vi "re_1.vi"(1 "wait_ms":u32=1000) -> (0 "timer_ms":u32)   [LabVIEW 2015, in "lv_mutex_shared_1.lvlib"]
uses:
  lv_mutex_shared_1.lvlib
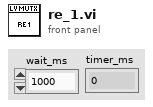
[diagram p1: front panel]
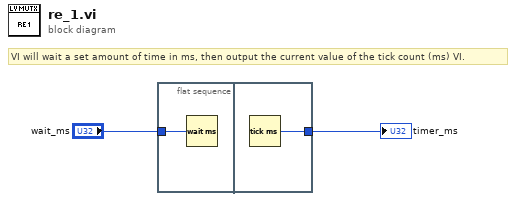
[diagram p0: block diagram]
diagram:
  # "VI will wait a set amount of time in ms, then output the current value of the tick count (ms) VI."
  n1 = flat-sequence {
    tunnel: "wait_ms" -> [w3]
    tunnel: [w4] -> w1
    frame #0 {
      n2 = Wait (ms)(milliseconds to wait=w3) -> ()  [unwired: 1 out]
    }
    frame #1 {
      n3 = Tick Count (ms)() -> (millisecond timer value=w4:u32)
    }
  }
  "timer_ms" <- w1
